vi "move path.vi"(1 "path selsction":T1, 2 "recy?":bool) -> (0 "path array":T2[](array[typedef]))   [LabVIEW 2019]
uses:
  ctl/path ctl.ctl
  ctl/position name.ctl
  ctl/path name.ctl
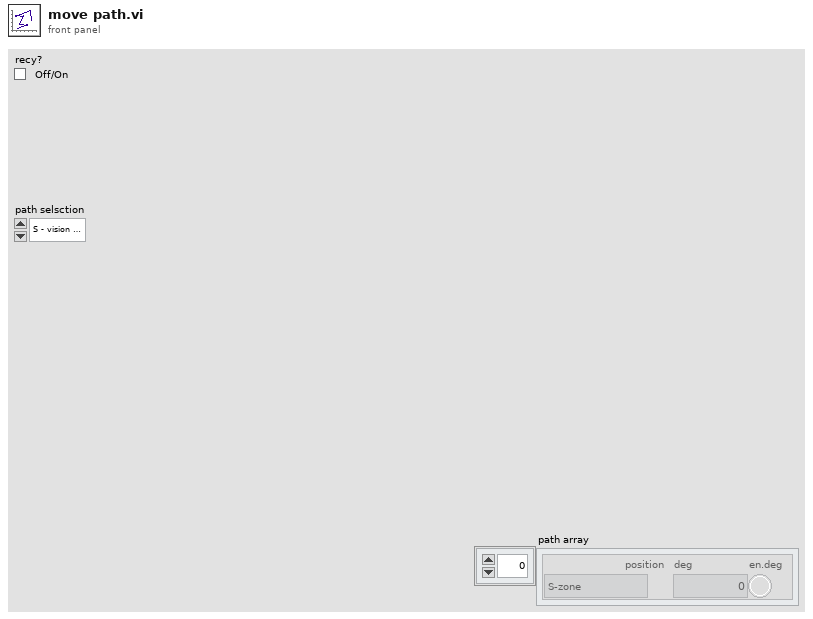
[diagram p1: front panel]
types:
  T1 = typedef "path name.ctl" = enum16{"S - vision board", "vision board - s out", "s out - room center", "room center - R1", "room center - R2", "room center - R3", "room center - R4", "room center - R5", "R1 - room center", "R2 - room center", "R3 - room center", "R4 - room center", "R5 - room center", "room center - S out", "S-out - recycle", "recycle - S-out", "S-out - s", "s - s-out", "board - box", "box - board", "S out - board", "R1 - R1 d", "R5d - R5", "R3.4-R3", "R3 - R3.2", "- align", "- align.5", "R2 - R2.d", "center align"}
  T2 = typedef "path ctl.ctl" = cluster{"position":T3, "deg":dbl, "en.deg":bool}
  T3 = typedef "position name.ctl" = enum16{"S-zone", "out S", "vision board-vision", "out box", "box catch", "room center", "room right", "room left", "R2", "R4", "only rotate", "out recy", "recycle", "R3", "near board", "box poxition", "R1", "R5", "R1-d", "R5-d", "R3.4", "align center.1", "align center.5", "R2-d", "R2-r", "far center"}
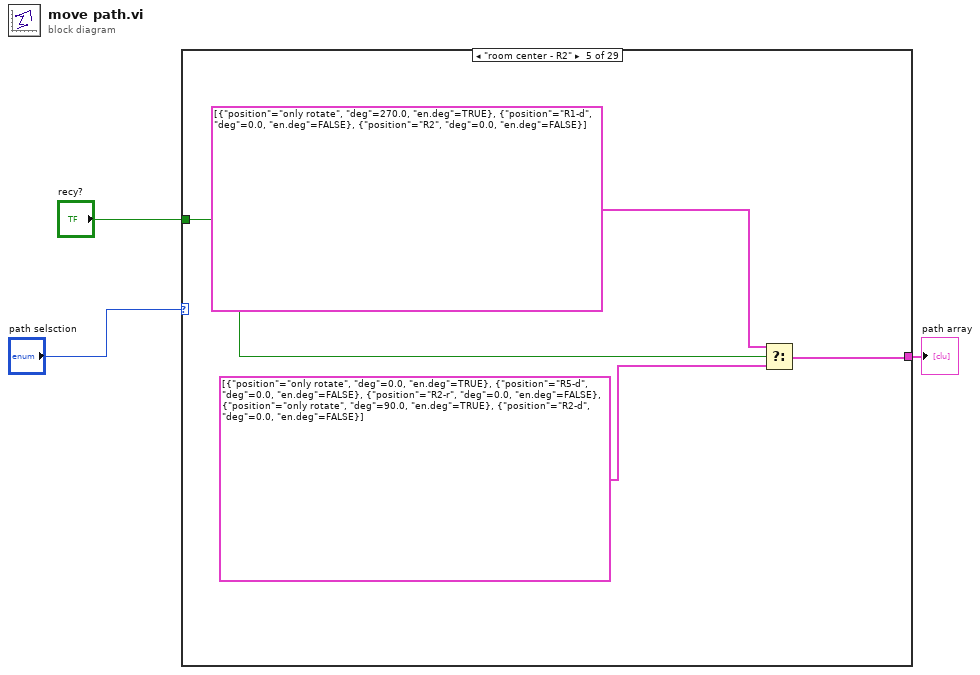
[diagram p0: block diagram]
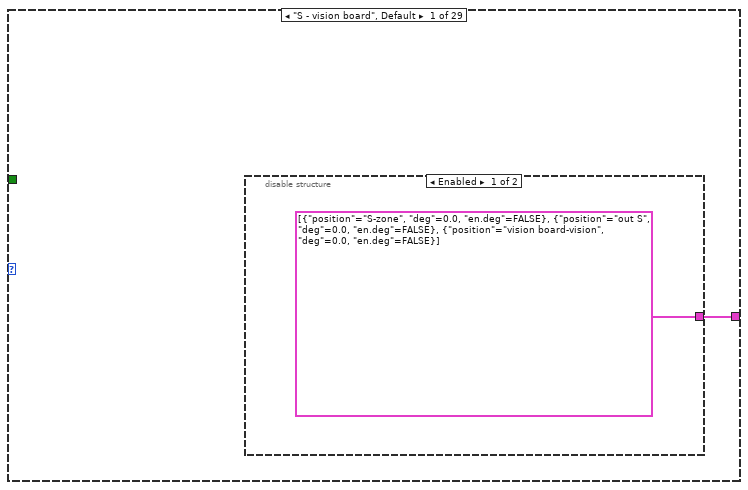
[diagram p2: hidden frame]
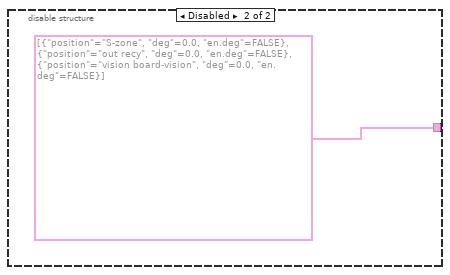
[diagram p3: hidden frame]
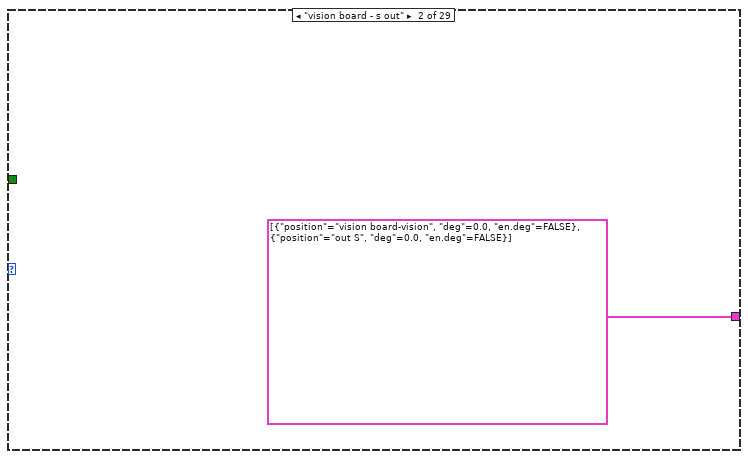
[diagram p4: hidden frame]
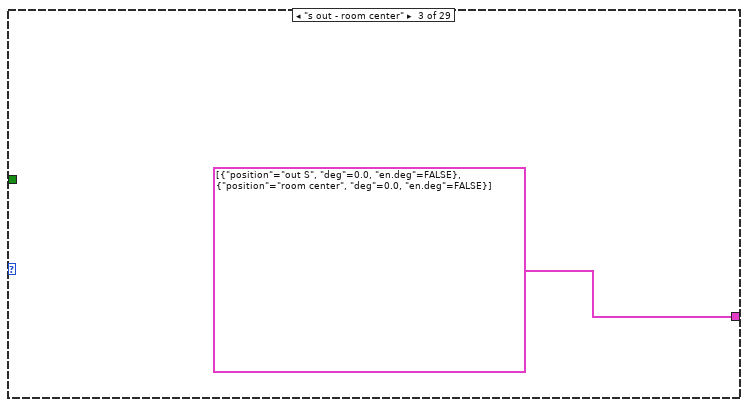
[diagram p5: hidden frame]
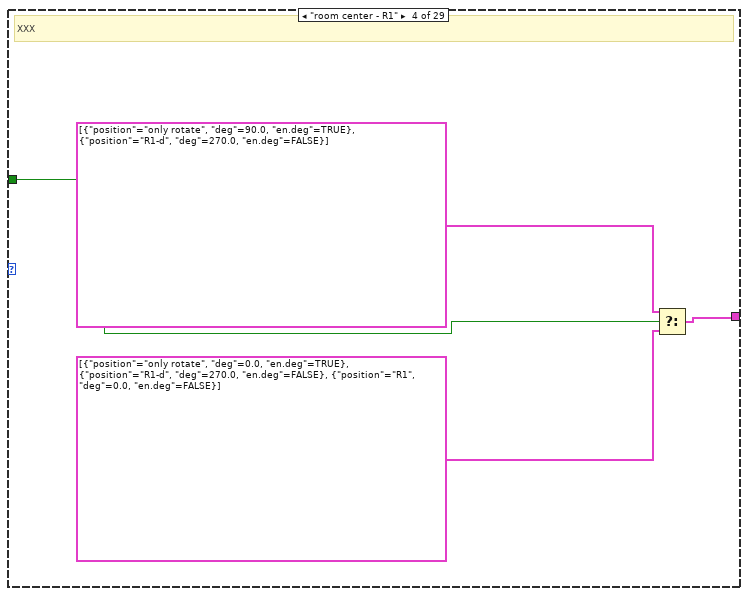
[diagram p6: hidden frame]
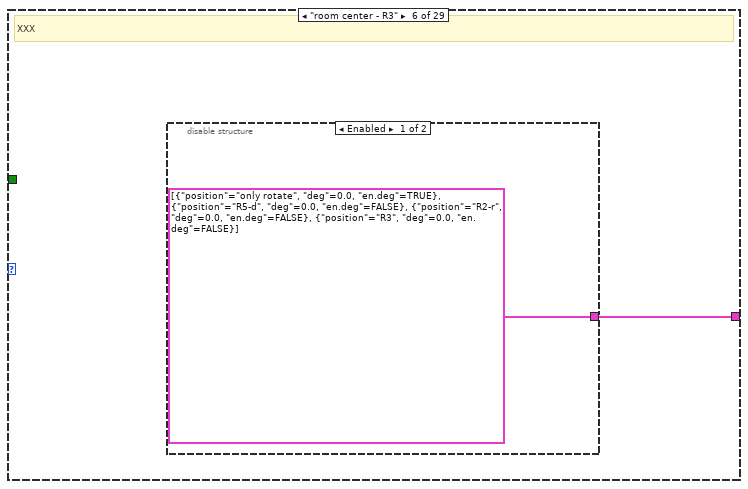
[diagram p7: hidden frame]
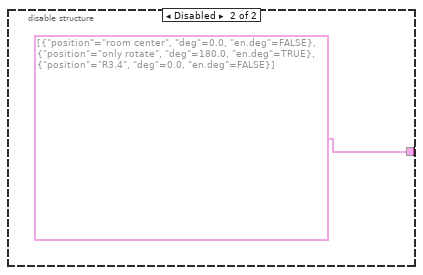
[diagram p8: hidden frame]
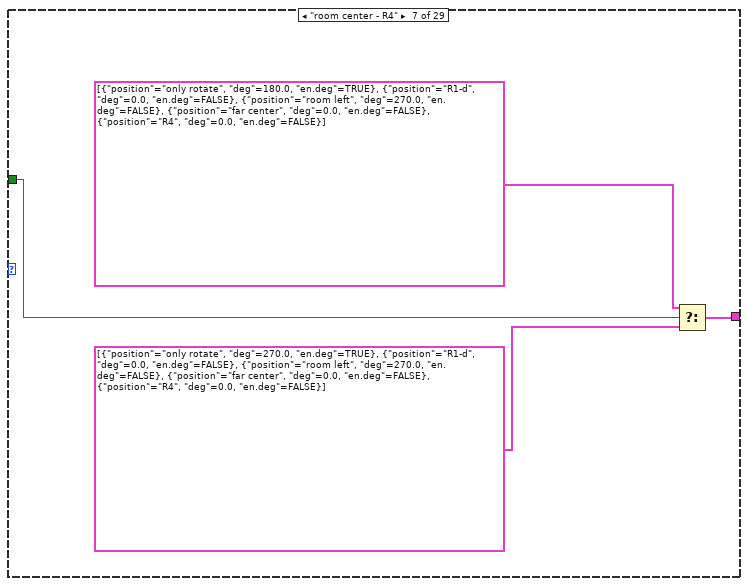
[diagram p9: hidden frame]
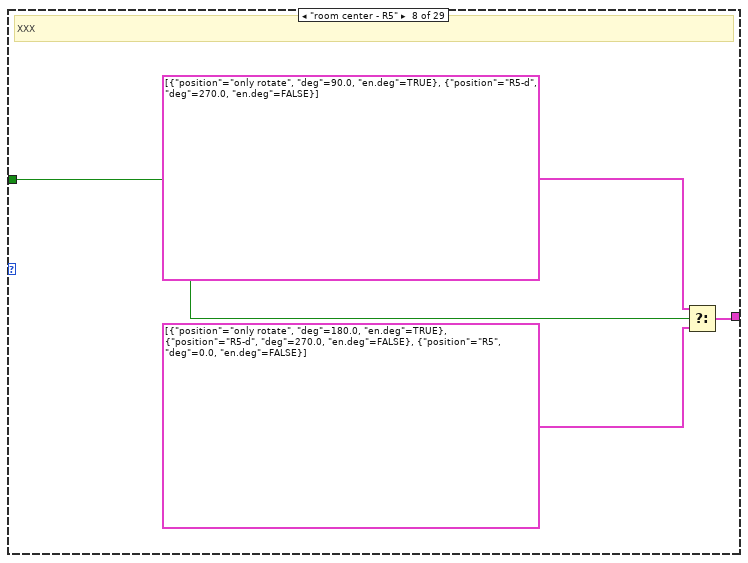
[diagram p10: hidden frame]
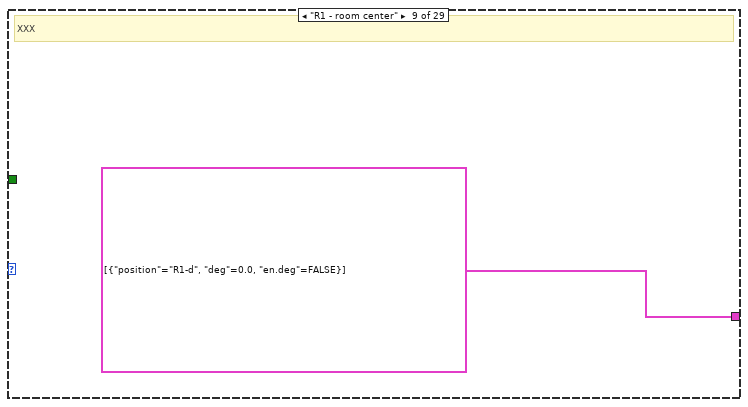
[diagram p11: hidden frame]
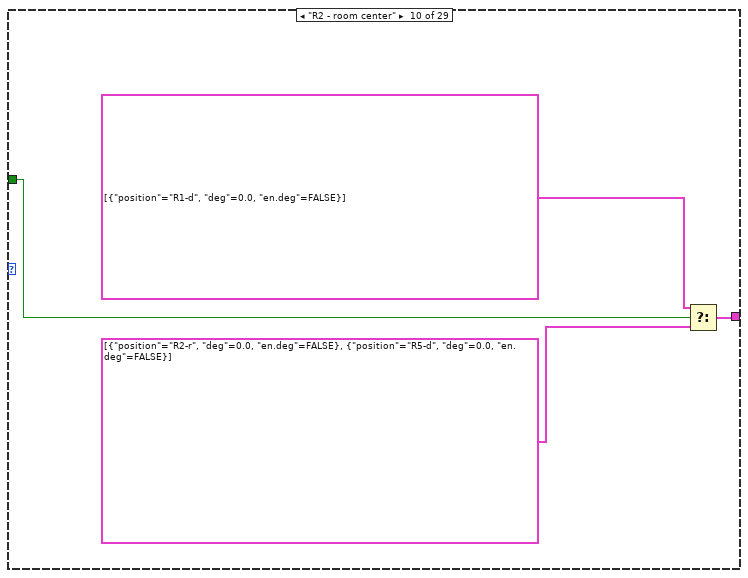
[diagram p12: hidden frame]
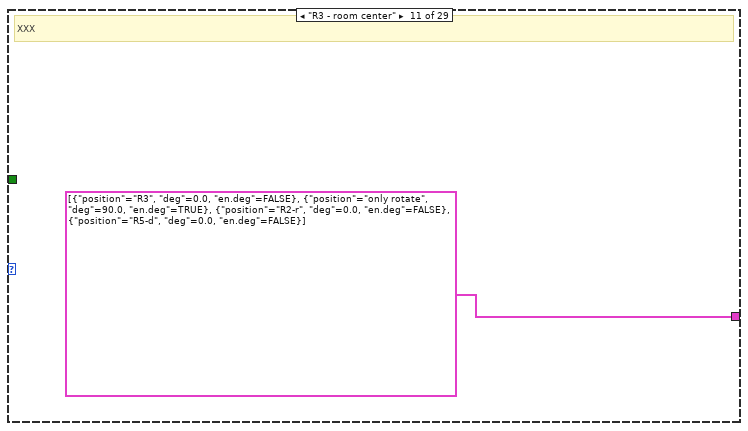
[diagram p13: hidden frame]
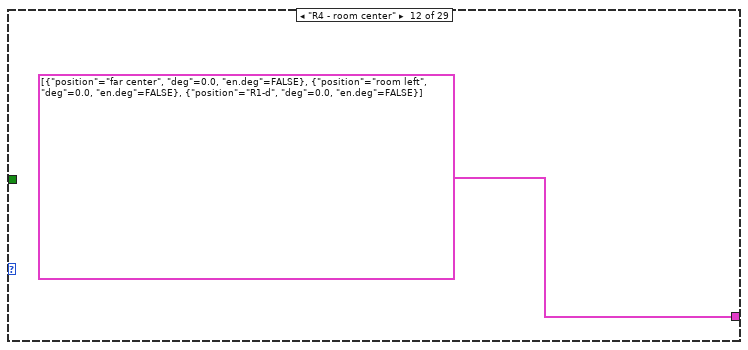
[diagram p14: hidden frame]
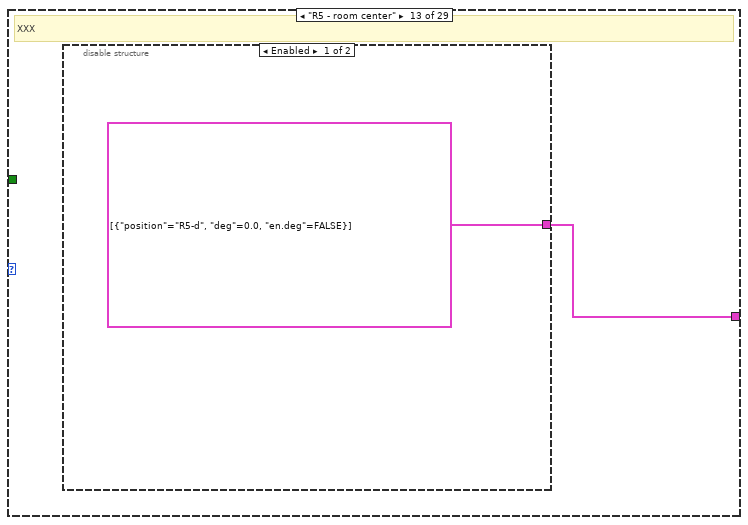
[diagram p15: hidden frame]
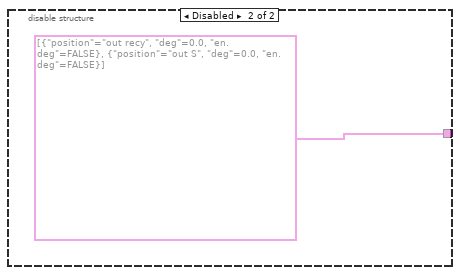
[diagram p16: hidden frame]
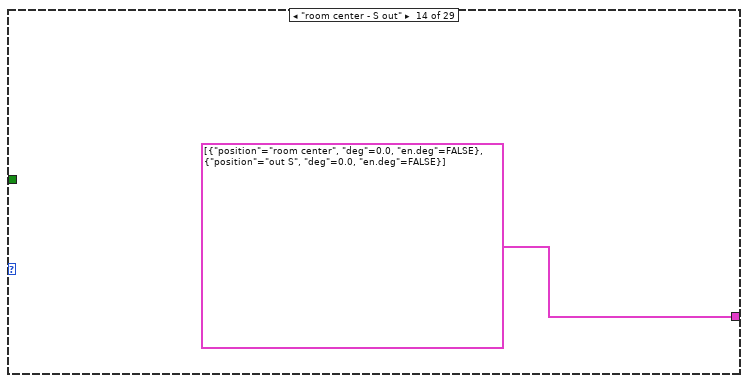
[diagram p17: hidden frame]
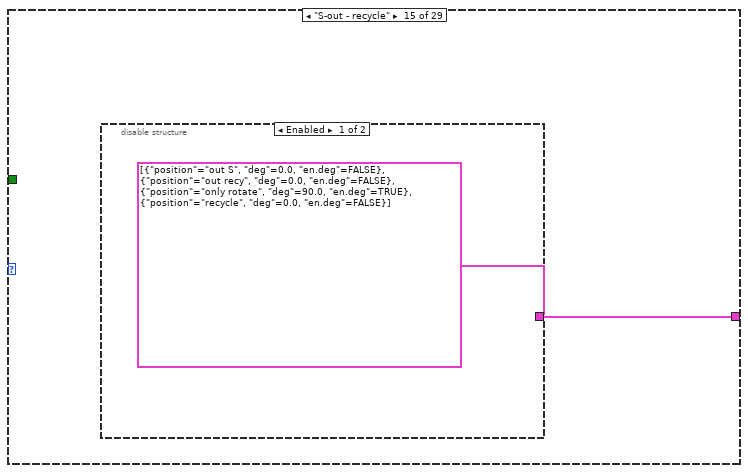
[diagram p18: hidden frame]
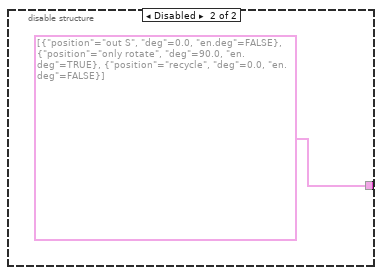
[diagram p19: hidden frame]
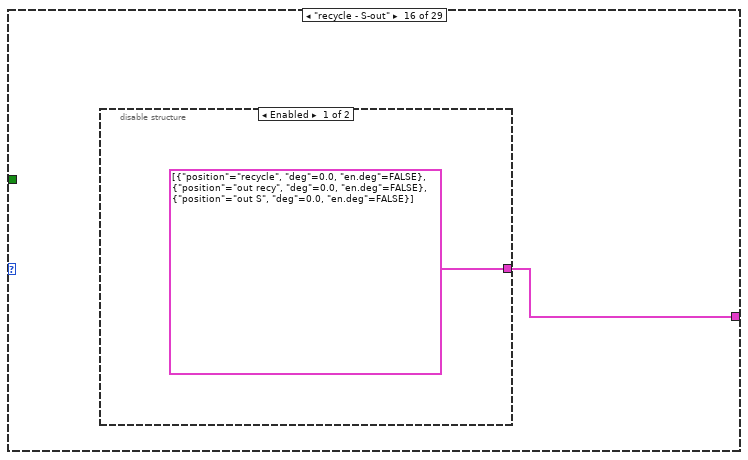
[diagram p20: hidden frame]
diagram:
  n1 = case shown="\"room center - R2\"" "path selsction" {
    tunnel: [w4 T2[] [{"position"=enum."vision board-vision", "deg"=0.0, "en.deg"=FALSE}, {"position"=enum."out S", "deg"=0.0, "en.deg"=FALSE}] ("Array") T2[] [{"position"=enum."out S", "deg"=0.0, "en.deg"=FALSE}, {"position"=enum."room center", "deg"=0.0, "en.deg"=FALSE}] ("Array") w11 w16 w17 w22 w26 T2[] [{"position"=enum."R1-d", "deg"=0.0, "en.deg"=FALSE}] ("Array") w31 T2[] [{"position"=enum."R3", "deg"=0.0, "en.deg"=FALSE}, {"position"=enum."only rotate", "deg"=90.0, "en.deg"=TRUE}, {"position"=enum."R2-r", "deg"=0.0, "en.deg"=FALSE}, {"position"=enum."R5-d", "deg"=0.0, "en.deg"=FALSE}] ("Array") T2[] [{"position"=enum."far center", "deg"=0.0, "en.deg"=FALSE}, {"position"=enum."room left", "deg"=0.0, "en.deg"=FALSE}, {"position"=enum."R1-d", "deg"=0.0, "en.deg"=FALSE}] ("Array") w35 T2[] [{"position"=enum."room center", "deg"=0.0, "en.deg"=FALSE}, {"position"=enum."out S", "deg"=0.0, "en.deg"=FALSE}] ("Array") w39 w42 w45 w48 T2[] [{"position"=enum."vision board-vision", "deg"=0.0, "en.deg"=FALSE}, {"position"=enum."near board", "deg"=0.0, "en.deg"=FALSE}, {"position"=enum."only rotate", "deg"=90.0, "en.deg"=TRUE}, {"position"=enum."box poxition", "deg"=0.0, "en.deg"=FALSE}] ("Array") T2[] [{"position"=enum."box poxition", "deg"=0.0, "en.deg"=FALSE}, {"position"=enum."near board", "deg"=0.0, "en.deg"=FALSE}, {"position"=enum."vision board-vision", "deg"=0.0, "en.deg"=FALSE}] ("Array") T2[] [{"position"=enum."out S", "deg"=0.0, "en.deg"=FALSE}, {"position"=enum."vision board-vision", "deg"=0.0, "en.deg"=FALSE}] ("Array") T2[] [{"position"=enum."room left", "deg"=0.0, "en.deg"=FALSE}, {"position"=enum."only rotate", "deg"=90.0, "en.deg"=TRUE}, {"position"=enum."R1-d", "deg"=0.0, "en.deg"=FALSE}] ("Array") w55 T2[] [{"position"=enum."R3.4", "deg"=0.0, "en.deg"=FALSE}, {"position"=enum."room center", "deg"=0.0, "en.deg"=FALSE}, {"position"=enum."only rotate", "deg"=270.0, "en.deg"=TRUE}, {"position"=enum."R3", "deg"=0.0, "en.deg"=FALSE}] ("Array") T2[] [{"position"=enum."R3.4", "deg"=0.0, "en.deg"=FALSE}, {"position"=enum."room center", "deg"=0.0, "en.deg"=FALSE}, {"position"=enum."only rotate", "deg"=0.0, "en.deg"=TRUE}, {"position"=enum."R3", "deg"=0.0, "en.deg"=FALSE}] ("Array") T2[] [{"position"=enum."align center.1", "deg"=0.0, "en.deg"=FALSE}, {"position"=enum."only rotate", "deg"=0.0, "en.deg"=TRUE}] ("Array") T2[] [{"position"=enum."align center.1", "deg"=0.0, "en.deg"=FALSE}, {"position"=enum."only rotate", "deg"=180.0, "en.deg"=TRUE}] ("Array") T2[] [{"position"=enum."R2-r", "deg"=0.0, "en.deg"=FALSE}, {"position"=enum."only rotate", "deg"=90.0, "en.deg"=TRUE}, {"position"=enum."R2-d", "deg"=0.0, "en.deg"=FALSE}] ("Array") T2[] [{"position"=enum."room center", "deg"=0.0, "en.deg"=FALSE}, {"position"=enum."only rotate", "deg"=270.0, "en.deg"=TRUE}] ("Array")] -> w2
    tunnel: "recy?" -> [_ _ _ w10 w14 _ w21 w25 _ w30 _ _ _ _ _ _ _ _ _ _ _ _ _ _ _ _ _ _ _]
    frame "S - vision board", Default {
      n2 = disable-structure shown="Enabled" {
        disable-tunnel: [T2[] [{"position"=enum."S-zone", "deg"=0.0, "en.deg"=FALSE}, {"position"=enum."out S", "deg"=0.0, "en.deg"=FALSE}, {"position"=enum."vision board-vision", "deg"=0.0, "en.deg"=FALSE}] ("Array") T2[] [{"position"=enum."S-zone", "deg"=0.0, "en.deg"=FALSE}, {"position"=enum."out recy", "deg"=0.0, "en.deg"=FALSE}, {"position"=enum."vision board-vision", "deg"=0.0, "en.deg"=FALSE}] ("Array")] -> w4
        frame Enabled {
        }
        frame Disabled {
        }
      }
    }
    frame "vision board - s out" {
    }
    frame "s out - room center" {
    }
    frame "room center - R1" {
      # "XXX"
      n3 = Select(t=T2[] [{"position"=enum."only rotate", "deg"=90.0, "en.deg"=TRUE}, {"position"=enum."R1-d", "deg"=270.0, "en.deg"=FALSE}] ("Array"), s=w10, f=T2[] [{"position"=enum."only rotate", "deg"=0.0, "en.deg"=TRUE}, {"position"=enum."R1-d", "deg"=270.0, "en.deg"=FALSE}, {"position"=enum."R1", "deg"=0.0, "en.deg"=FALSE}] ("Array")) -> (s? t:f=w11:T2[])
    }
    frame "room center - R2" {
      n4 = Select(t=T2[] [{"position"=enum."only rotate", "deg"=270.0, "en.deg"=TRUE}, {"position"=enum."R1-d", "deg"=0.0, "en.deg"=FALSE}, {"position"=enum."R2", "deg"=0.0, "en.deg"=FALSE}] ("Array"), s=w14, f=T2[] [{"position"=enum."only rotate", "deg"=0.0, "en.deg"=TRUE}, {"position"=enum."R5-d", "deg"=0.0, "en.deg"=FALSE}, {"position"=enum."R2-r", "deg"=0.0, "en.deg"=FALSE}, {"position"=enum."only rotate", "deg"=90.0, "en.deg"=TRUE}, {"position"=enum."R2-d", "deg"=0.0, "en.deg"=FALSE}] ("Array")) -> (s? t:f=w16:T2[])
    }
    frame "room center - R3" {
      # "XXX"
      n5 = disable-structure shown="Enabled" {
        disable-tunnel: [T2[] [{"position"=enum."only rotate", "deg"=0.0, "en.deg"=TRUE}, {"position"=enum."R5-d", "deg"=0.0, "en.deg"=FALSE}, {"position"=enum."R2-r", "deg"=0.0, "en.deg"=FALSE}, {"position"=enum."R3", "deg"=0.0, "en.deg"=FALSE}] ("Array") T2[] [{"position"=enum."room center", "deg"=0.0, "en.deg"=FALSE}, {"position"=enum."only rotate", "deg"=180.0, "en.deg"=TRUE}, {"position"=enum."R3.4", "deg"=0.0, "en.deg"=FALSE}] ("Array")] -> w17
        frame Enabled {
        }
        frame Disabled {
        }
      }
    }
    frame "room center - R4" {
      n6 = Select(t=T2[] [{"position"=enum."only rotate", "deg"=180.0, "en.deg"=TRUE}, {"position"=enum."R1-d", "deg"=0.0, "en.deg"=FALSE}, {"position"=enum."room left", "deg"=270.0, "en.deg"=FALSE}, {"position"=enum."far center", "deg"=0.0, "en.deg"=FALSE}, {"position"=enum."R4", "deg"=0.0, "en.deg"=FALSE}] ("Array"), s=w21, f=T2[] [{"position"=enum."only rotate", "deg"=270.0, "en.deg"=TRUE}, {"position"=enum."R1-d", "deg"=0.0, "en.deg"=FALSE}, {"position"=enum."room left", "deg"=270.0, "en.deg"=FALSE}, {"position"=enum."far center", "deg"=0.0, "en.deg"=FALSE}, {"position"=enum."R4", "deg"=0.0, "en.deg"=FALSE}] ("Array")) -> (s? t:f=w22:T2[])
    }
    frame "room center - R5" {
      # "XXX"
      n7 = Select(t=T2[] [{"position"=enum."only rotate", "deg"=90.0, "en.deg"=TRUE}, {"position"=enum."R5-d", "deg"=270.0, "en.deg"=FALSE}] ("Array"), s=w25, f=T2[] [{"position"=enum."only rotate", "deg"=180.0, "en.deg"=TRUE}, {"position"=enum."R5-d", "deg"=270.0, "en.deg"=FALSE}, {"position"=enum."R5", "deg"=0.0, "en.deg"=FALSE}] ("Array")) -> (s? t:f=w26:T2[])
    }
    frame "R1 - room center" {
      # "XXX"
    }
    frame "R2 - room center" {
      n8 = Select(t=T2[] [{"position"=enum."R1-d", "deg"=0.0, "en.deg"=FALSE}] ("Array"), s=w30, f=T2[] [{"position"=enum."R2-r", "deg"=0.0, "en.deg"=FALSE}, {"position"=enum."R5-d", "deg"=0.0, "en.deg"=FALSE}] ("Array")) -> (s? t:f=w31:T2[])
    }
    frame "R3 - room center" {
      # "XXX"
    }
    frame "R4 - room center" {
    }
    frame "R5 - room center" {
      # "XXX"
      n9 = disable-structure shown="Enabled" {
        disable-tunnel: [T2[] [{"position"=enum."R5-d", "deg"=0.0, "en.deg"=FALSE}] ("Array") T2[] [{"position"=enum."out recy", "deg"=0.0, "en.deg"=FALSE}, {"position"=enum."out S", "deg"=0.0, "en.deg"=FALSE}] ("Array")] -> w35
        frame Enabled {
        }
        frame Disabled {
        }
      }
    }
    frame "room center - S out" {
    }
    frame "S-out - recycle" {
      n10 = disable-structure shown="Enabled" {
        disable-tunnel: [T2[] [{"position"=enum."out S", "deg"=0.0, "en.deg"=FALSE}, {"position"=enum."out recy", "deg"=0.0, "en.deg"=FALSE}, {"position"=enum."only rotate", "deg"=90.0, "en.deg"=TRUE}, {"position"=enum."recycle", "deg"=0.0, "en.deg"=FALSE}] ("Array") T2[] [{"position"=enum."out S", "deg"=0.0, "en.deg"=FALSE}, {"position"=enum."only rotate", "deg"=90.0, "en.deg"=TRUE}, {"position"=enum."recycle", "deg"=0.0, "en.deg"=FALSE}] ("Array")] -> w39
        frame Enabled {
        }
        frame Disabled {
        }
      }
    }
    frame "recycle - S-out" {
      n11 = disable-structure shown="Enabled" {
        disable-tunnel: [T2[] [{"position"=enum."recycle", "deg"=0.0, "en.deg"=FALSE}, {"position"=enum."out recy", "deg"=0.0, "en.deg"=FALSE}, {"position"=enum."out S", "deg"=0.0, "en.deg"=FALSE}] ("Array") T2[] [{"position"=enum."recycle", "deg"=0.0, "en.deg"=FALSE}, {"position"=enum."out S", "deg"=0.0, "en.deg"=FALSE}] ("Array")] -> w42
        frame Enabled {
        }
        frame Disabled {
        }
      }
    }
    frame "S-out - s" {
      n12 = disable-structure shown="Enabled" {
        disable-tunnel: [T2[] [{"position"=enum."out S", "deg"=0.0, "en.deg"=FALSE}, {"position"=enum."only rotate", "deg"=0.0, "en.deg"=TRUE}, {"position"=enum."S-zone", "deg"=0.0, "en.deg"=FALSE}] ("Array") T2[] [{"position"=enum."out S", "deg"=0.0, "en.deg"=FALSE}, {"position"=enum."out recy", "deg"=0.0, "en.deg"=FALSE}, {"position"=enum."only rotate", "deg"=0.0, "en.deg"=TRUE}, {"position"=enum."S-zone", "deg"=0.0, "en.deg"=FALSE}] ("Array")] -> w45
        frame Enabled {
        }
        frame Disabled {
        }
      }
    }
    frame "s - s-out" {
      n13 = disable-structure shown="Enabled" {
        disable-tunnel: [T2[] [{"position"=enum."S-zone", "deg"=0.0, "en.deg"=FALSE}, {"position"=enum."out S", "deg"=0.0, "en.deg"=FALSE}] ("Array") T2[] [{"position"=enum."S-zone", "deg"=0.0, "en.deg"=FALSE}, {"position"=enum."out recy", "deg"=0.0, "en.deg"=FALSE}, {"position"=enum."out S", "deg"=0.0, "en.deg"=FALSE}] ("Array")] -> w48
        frame Enabled {
        }
        frame Disabled {
        }
      }
    }
    frame "board - box" {
    }
    frame "box - board" {
    }
    frame "S out - board" {
    }
    frame "R1 - R1 d" {
    }
    frame "R5d - R5" {
      n14 = disable-structure shown="Enabled" {
        disable-tunnel: [T2[] [{"position"=enum."R5-d", "deg"=0.0, "en.deg"=FALSE}, {"position"=enum."room right", "deg"=0.0, "en.deg"=FALSE}, {"position"=enum."only rotate", "deg"=180.0, "en.deg"=TRUE}, {"position"=enum."R5", "deg"=0.0, "en.deg"=FALSE}] ("Array") T2[] [{"position"=enum."out recy", "deg"=0.0, "en.deg"=FALSE}, {"position"=enum."out S", "deg"=0.0, "en.deg"=FALSE}, {"position"=enum."only rotate", "deg"=270.0, "en.deg"=TRUE}, {"position"=enum."out recy", "deg"=0.0, "en.deg"=FALSE}] ("Array")] -> w55
        frame Enabled {
        }
        frame Disabled {
        }
      }
    }
    frame "R3.4-R3" {
    }
    frame "R3 - R3.2" {
    }
    frame "- align" {
    }
    frame "- align.5" {
    }
    frame "R2 - R2.d" {
    }
    frame "center align" {
    }
  }
  "path array" <- w2
